vi "About.vi"(8 "error in (no error)":errorcluster, 11 "Calling VI in":refnum<vi>) -> (0 "error out":errorcluster)   [LabVIEW 2020, in "MacroAssert.lvlib"]
doc: "Displays a window that shows various information about the tool."
uses:
  MacroAssert.lvlib
panel:
  out "Version Info":string="version #.#.#.# - Month DD, YYYY"
  # "MacroAssert"
  # "by Andrew Casalenuovo"
  # "VIPM Package: https://www.vipm.io/package/redhawk_lib_macroassert/"
  # "GitHub Repository: https://github.com/FireFist-Redhawk/MacroAssert"
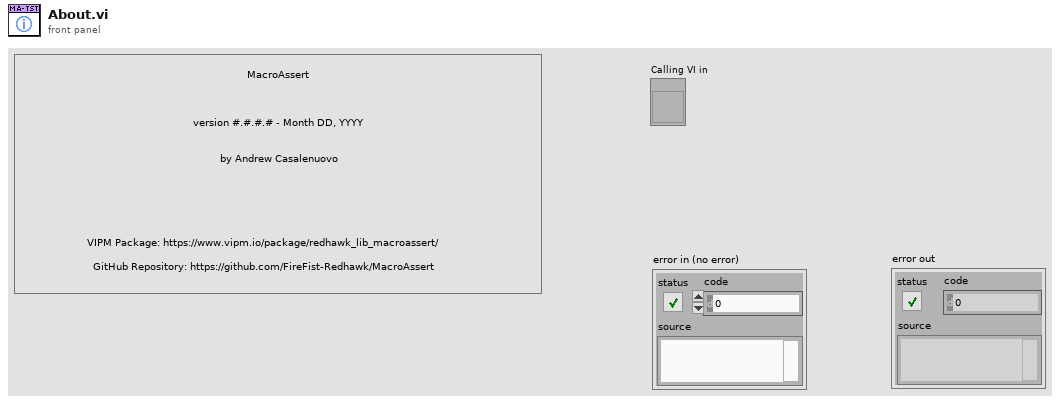
[diagram p1: front panel]
types:
  T1 = enum32{"Invalid", "Standard", "Closed", "Hidden", "Minimized", "Maximized"}
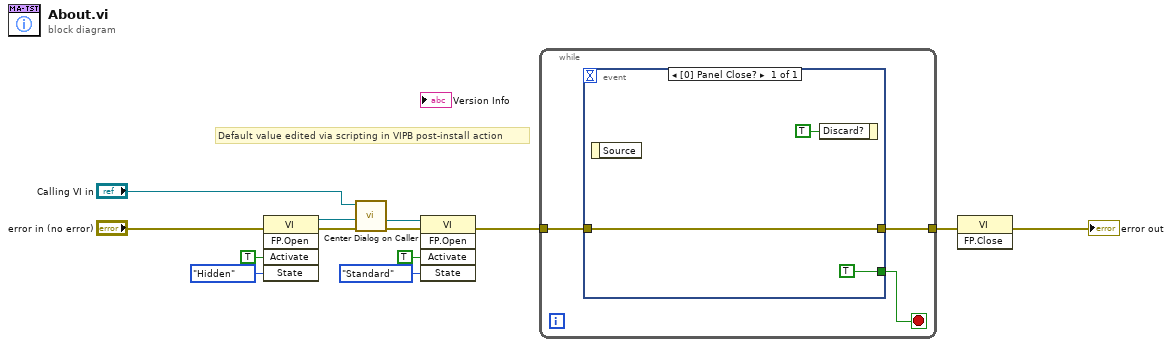
[diagram p0: block diagram]
diagram:
  # "Default value edited via scripting in VIPB post-install action"
  n1 = invoke class="VI" method="FP.Open"(error in="error in (no error)", "Activate"=TRUE ("Activate?"), "State"=T1."Hidden") -> (reference out=w2:refnum<vi>, error out=w5:errorcluster)  [unwired: 2 in, 3 out]
  n2 = call "Center Dialog on Caller.vi"("error in (no error)"=w5, "Dialog VI"=w2, "Calling VI in"="Calling VI in") -> ("error out"=w4:errorcluster, "Dialog VI out"=w1:refnum<vi>)  [unwired: 7 in]
  n3 = invoke class="VI" method="FP.Open"(reference=w1, error in=w4, "Activate"=TRUE ("Activate?"), "State"=T1."Standard") -> (error out=w11:errorcluster)  [unwired: 1 in, 4 out]
  n4 = while {
    tunnel: [w15] -> w13
    tunnel: w11 -> [w14]
    stop <- w16 stop-if-true
    n5 = event shown="[0] Panel Close?" {
      selector: _ -> [_]
      dyn-events: _ -> [_]
      timeout: _ -> [_]
      tunnel: [TRUE] -> w16
      tunnel: [w17] -> w15
      tunnel: w14 -> [w17]
      event Panel Close? {
        n6 = event-data() -> ()  [unwired: 1 in, 1 out]
        n7 = event-data("Discard?"=TRUE) -> ()  [unwired: 1 in, 1 out]
      }
    }
  }
  n8 = invoke class="VI" method="FP.Close"(error in=w13) -> (error out=→"error out":errorcluster)  [unwired: 2 in, 2 out]
